vi "Wait.vi"(8 "error in (no error)":errorcluster, 10 "Timeout in ms (0)":i32, 11 "Sequencer in":refnum<class "Sequencer.lvclass">) -> (0 "error out":errorcluster, 1 "Timed out?":bool, 3 "Sequencer out":refnum<class "Sequencer.lvclass">)   [LabVIEW 2020, in "Sequencer.lvlib" / "Sequencer.lvclass"]
doc: "Execute the Sequencer Core Wait method."
uses:
  Sequencer.lvclass
  Sequencer.lvclass/Sequencer.ctl
  Sequencer Core/Sequencer Core.lvclass/Sequencer Core.ctl
  PPL/HDH.Data.Generic.lvlibp/Synchronization/Notifier/Wait Single.vi
  Sequencer Core/Sequencer Core.lvclass
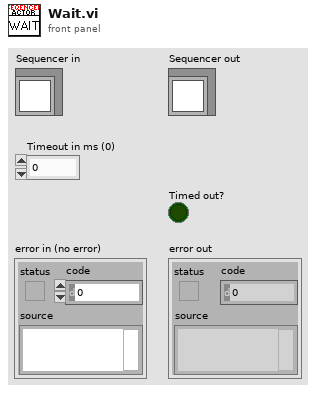
[diagram p1: front panel]
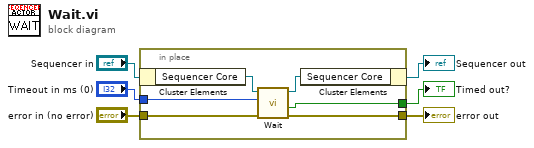
[diagram p0: block diagram]
diagram:
  n1 = in-place {
    in-place-border: "error in (no error)" -> [w10]
    in-place-border: [w9] -> w5
    in-place-border: "Timeout in ms (0)" -> [w8]
    in-place-border: [w7] -> w2
    n2 = in-place-cluster #1("Sequencer in") -> ("Sequencer Core"=w12:refnum<class "Sequencer Core.lvclass">)
    n3 = call "Wait.vi"("error in (no error)"=w10, "Timeout in ms (0)"=w8, "Sequencer Core in"=w12) -> ("error out"=w9:errorcluster, "Timed out?"=w7:bool, "Sequencer Core out"=w11:refnum<class "Sequencer Core.lvclass">)  [unwired: 6 in]
    n4 = in-place-cluster #1("Sequencer Core"=w11) -> (→"Sequencer out":refnum<class "Sequencer.lvclass">)
  }
  "error out" <- w5
  "Timed out?" <- w2
